vi "Reset.vi"(8 "error in (no error)":errorcluster, 11 "NhRegenGridSim in":refnum<class "NHRGridSim.lvclass">) -> (0 "error out":errorcluster, 3 "NhRegenGridSim out":refnum<class "NHRGridSim.lvclass">)   [LabVIEW 2018, in "AcPwrPlugins.lvlib" / "NHRGridSim.lvclass"]
doc: "This VI resets the instrument to <B>original power on configuration</B>. Does not clear Enable register for Standard Summary Status or Standard Event Registers. Does not clear the output queue. Does not clear the power-on-status-clear flag."
uses:
  NHRGridSim.lvclass
  <instrlib>/NH Research 9400 Series/NH Research 9400 Series.lvlib
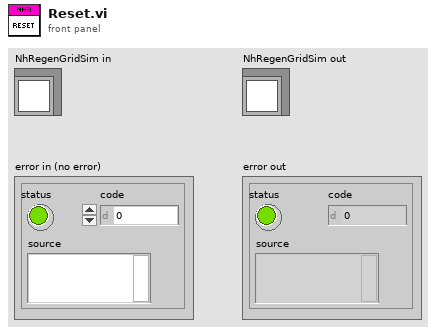
[diagram p1: front panel]
types:
  T1 = typedef "AcPwrPlugins.lvlib/NHRGridSim.lvclass/Device(s)Settings.ctl" = cluster{"MeasName":string, "Instr1":T2, "Instr2":T2, "Instr3":T2, "Handle":string, "Reset":bool, "Mode":T9, "ID Query":bool, "Connected":bool}
  T2 = typedef "AcPwrPlugins.lvlib/NHRGridSim.lvclass/NHRGrid_InstrumentCluster_Tabs.ctl" = cluster{"Name":string, "Vout (V)":dbl, "VType":string, "Phases":T3, "FreqOut (Hz)":dbl, "Aperture (cycles)":i32, "Configure Instrument":T4, "AC Wave Shape":T5, "Ranges":T6, "Safety Trips":T7, "Slew Rates":T8}
  T3 = typedef "AcPwrPlugins.lvlib/NHRGridSim.lvclass/NHRGrid_Phases_Tabs.ctl" = cluster{"A-Volts (V)":dbl, "B-Volts (V)":dbl, "C-Volts (V)":dbl, "Change at (Deg)":i32, "B-Angle (Deg)":i32, "C-Angle (Deg)":i32}
  T4 = typedef "AcPwrPlugins.lvlib/NHRGridSim.lvclass/NHRGrid_Configure_Tabs.ctl" = u16
  T5 = typedef "AcPwrPlugins.lvlib/NHRGridSim.lvclass/NHRGrid_WaveShape_Tabs.ctl" = u16
  T6 = typedef "AcPwrPlugins.lvlib/NHRGridSim.lvclass/NHRGrid_Ranges_Tabs.ctl" = cluster{"Voltage (V)":u16, "Current (A)":u16}
  T7 = typedef "AcPwrPlugins.lvlib/NHRGridSim.lvclass/NHRGrid_SafetyTrips_Tabs.ctl" = cluster{"Vmax (V)":dbl, "Vmin (V)":dbl, "Vmax Time (s)":dbl, "Vmin Time (s)":dbl, "Imax Source (A)":dbl, "Imax Sink (A)":dbl, "I Src Time (s)":dbl, "I Snk Time (s)":dbl, "Pmax Source (W)":dbl, "Pmax Sink (W)":dbl, "P Src Time (s)":dbl, "P Snk Time (s)":dbl, "Abs Volt Peak":dbl, "Enable Vpk":bool, "Abs Curr Peak":dbl, "Enable Ipk":bool}
  T8 = typedef "AcPwrPlugins.lvlib/NHRGridSim.lvclass/NHRGrid_SlewRates_Tabs.ctl" = cluster{"Voltage (V/s)":dbl, "Current (A/s)":dbl, "Power (W/s)":dbl, "Frequency (Hz/s)":dbl, "Phase Angle (Deg/s)":dbl}
  T9 = typedef "AcPwrPlugins.lvlib/NHRGridSim.lvclass/NHRGrid_Modes.ctl" = u8
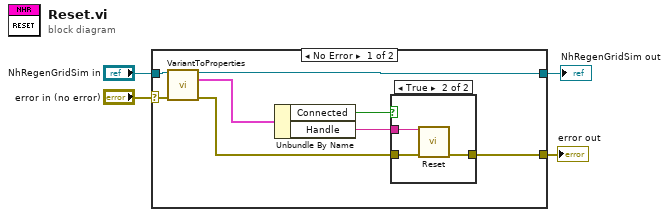
[diagram p0: block diagram]
diagram:
  n1 = case shown="No Error" "error in (no error)" {
    selector: "error in (no error)" -> [w11 w17]
    tunnel: "NhRegenGridSim in" -> [w10 w18]
    tunnel: [w9 w18] -> w2
    tunnel: [w12 w17] -> w1
    frame No Error {
      n2 = call "VariantToProperties.vi"("NHRGridSim in"=w10, "error in (no error)"=w11) -> ("NHRGridSim out"=w9:refnum<class "NHRGridSim.lvclass">, "Device(s)Settings"=w7:T1, "error out"=w8:errorcluster)  [unwired: 8 in, 3 out]
      n3 = Unbundle By Name(w7) -> ("Connected"=w5:bool, "Handle"=w6:string)
      n4 = case shown="True" w5 {
        tunnel: w6 -> [_ w16]
        tunnel: w8 -> [w13 w15]
        tunnel: [w13 w14] -> w12
        frame False {
        }
        frame True {
          n5 = call <instrlib>:"Reset.vi"("VISA resource name"=w16, "error in (no error)"=w15) -> ("error out"=w14:errorcluster)  [unwired: 12 in, 1 out]
        }
      }
    }
    frame Error {
    }
  }
  "error out" <- w1
  "NhRegenGridSim out" <- w2
